vi "draw3.vi"(0 "new position":cluster{"x":i16, "y":i16}, 1 "L 1":dbl(slide)=80.0 scale=0.0..200.0, 2 "L 2":dbl(slide)=80.0 scale=0.0..200.0, 3 "Angle1":dbl(knob)=-45.83837436417874 scale=-90.0..90.0, 4 "Angle 2":dbl(knob)=-72.06882847083946 scale=-90.0..90.0, 5 "input pic in loop":picture, 7 "bias":dbl) -> (14 "end effector":cluster{dbl, dbl}={159.01647214211073, 1.9100783062530127} {"?" format="%.1f"; "?" format="%#.1f"}, 15 "mag":dbl, 16 "angle":dbl, 17 "2D Picture":picture, 18 "shift pic":picture)   [LabVIEW 2024]
panel:
  out "angle3":dbl
  in  "bias 2":dbl
  in  "L 3":dbl(slide)=80.0 scale=0.0..200.0
  # "A 2"
  # "L1"
  # "L2"
  # "A 1"
  # "mm"
  # "mm"
  # "mm"
  # "mm"
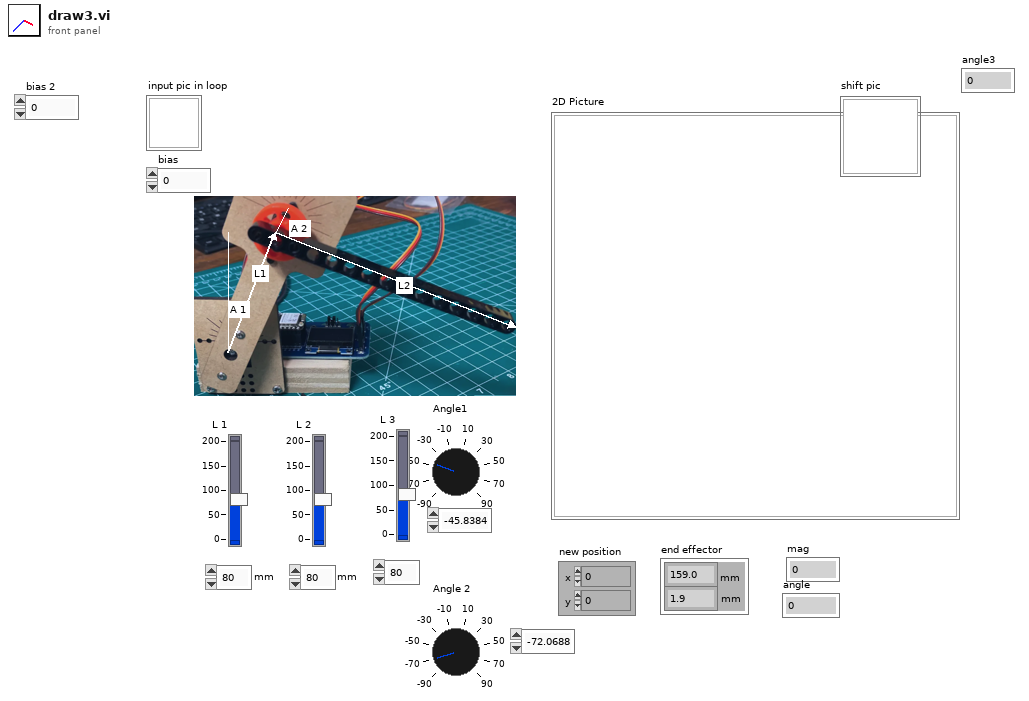
[diagram p1: front panel]
types:
  T1 = cluster{"Width":u16, "Style":enum32{"Solid", "Dash", "Dot", "DashDot", "DashDotDot"}}
  T2 = typedef "imagedata.ctl" = cluster{"image type":i32, "image depth":i32, "image":u8[], "mask":u8[], "colors":u32[], "Rectangle":cluster{"left":i16, "top":i16, "right":i16, "bottom":i16}}
  T3 = cluster{"left":i16, "top":i16, "right":i16, "bottom":i16}
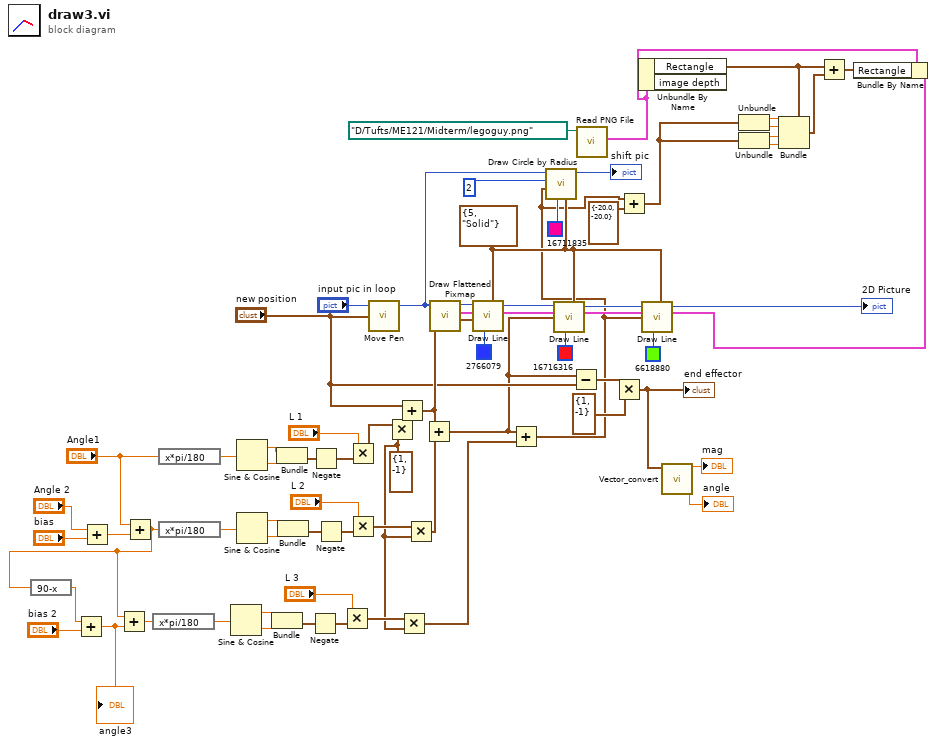
[diagram p0: block diagram]
diagram:
  w25 = cluster{"x":i16, "y":i16} {"x"=1, "y"=-1} ("new position")
  w21 = T1 {"Width"=5, "Style"=enum."Solid"} ("pen")
  n1 = Add(x="Angle 2", y="bias") -> (x+y=w27:dbl)
  n2 = Add(x="Angle1", y=w27) -> (x+y=w18:dbl)
  n3 = expression code="90-x"(w18) -> (w20:dbl)
  n4 = Add(x=w20, y="bias 2") -> (x+y=w29:dbl)
  "angle3" <- w29
  n5 = Add(x=w18, y=w29) -> (x+y=w34:dbl)
  n6 = expression code="x*pi/180"(w34) -> (w35:dbl)
  n7 = expression code="x*pi/180"("Angle1") -> (w68:dbl)
  n8 = expression code="x*pi/180"(w18) -> (w65:dbl)
  n9 = Sine & Cosine(0:w35) -> (1:w32:dbl, 2:w31:dbl)
  n10 = Sine & Cosine(0:w68) -> (1:w55:dbl, 2:w54:dbl)
  n11 = Sine & Cosine(0:w65) -> (1:w52:dbl, 2:w51:dbl)
  n12 = Bundle(w32, w31) -> (w36:cluster{dbl, dbl})  [unwired: 1 in]
  n13 = Bundle(w55, w54) -> (w67:cluster{dbl, dbl})  [unwired: 1 in]
  n14 = Bundle(w52, w51) -> (w66:cluster{dbl, dbl})  [unwired: 1 in]
  n15 = Negate(x=w36) -> (-x=w30:cluster{dbl, dbl})
  n16 = Negate(x=w67) -> (-x=w53:cluster{dbl, dbl})
  n17 = Negate(x=w66) -> (-x=w50:cluster{dbl, dbl})
  n18 = Multiply(x="L 3", y=w30) -> (x*y=w26:cluster{dbl, dbl})
  n19 = Multiply(x="L 1", y=w53) -> (x*y=w40:cluster{dbl, dbl})
  n20 = Multiply(x="L 2", y=w50) -> (x*y=w37:cluster{dbl, dbl})
  n21 = call <vilib>:"Move Pen.vi"("new position"="new position", "picture"="input pic in loop") -> ("new picture"=w5:picture)  [unwired: 3 in]
  n22 = Multiply(x=w40, y=w25) -> (x*y=w39:cluster{dbl, dbl})
  n23 = Add(x="new position", y=w39) -> (x+y=w63:cluster{dbl, dbl})
  n24 = Multiply(x=w26, y=w25) -> (x*y=w24:cluster{dbl, dbl})
  n25 = Multiply(x=w37, y=w25) -> (x*y=w38:cluster{dbl, dbl})
  n26 = Add(x=w38, y=w63) -> (x+y=w19:cluster{dbl, dbl})
  n27 = Add(x=w19, y=w24) -> (x+y=w3:cluster{dbl, dbl})
  n28 = call <vilib>:"Draw Circle by Radius.vi"("pen"=w21, "color(black)"=u32 16711835, "pixel center"=w3, "radius"=u16 2 ("Width"), "picture"=w5) -> ("new picture"=→"shift pic":picture)  [unwired: 6 in]
  n29 = Subtract(x=w19, y="new position") -> (x-y=w58:cluster{dbl, dbl})
  n30 = call <vilib>:"Read PNG File.vi"("path to PNG file"=path "D:/Tufts/ME121/Midterm/legoguy.png") -> ("image data"=w10:T2)  [unwired: 8 in, 2 out]
  n31 = Multiply(x=w58, y=cluster{"x":i16, "y":i16} {"x"=1, "y"=-1} ("new position")) -> (x*y=w49:cluster{dbl, dbl})
  "end effector" <- w49
  n32 = Add(x=w3, y=cluster{dbl, dbl} {-20.0, -20.0} ("x+y")) -> (x+y=w1:cluster{dbl, dbl})
  n33 = Unbundle By Name(w10) -> ("Rectangle"=w7:T3)  [unwired: 1 out]
  n34 = call "Vector_convert.vi"("x,y"=w49) -> ("angle"=→"angle":dbl, "mag"=→"mag":dbl)  [unwired: 9 in]
  n35 = Unbundle(w1) -> (w16:dbl, w15:dbl)
  n36 = Unbundle(w1) -> (w14:dbl, w13:dbl)
  n37 = Bundle(cluster=w7, "left"=w16, "top"=w15, "right"=w14, "bottom"=w13) -> (w8:T3)
  n38 = Add(x=w7, y=w8) -> (x+y=w9:T3)
  n39 = Bundle By Name(cluster=w10, "Rectangle"=w9) -> (w12:T2)
  n40 = call "Draw Flattened Pixmap.vi"("image data"=w12, "picture"=w5) -> ("new picture"=w4:picture)  [unwired: 7 in]
  n41 = call <vilib>:"Draw Line.vi"("picture"=w4, "end point"=w63, "color(black)"=u32 2766079, "pen"=w21) -> ("new picture"=w64:picture)  [unwired: 5 in]
  n42 = call <vilib>:"Draw Line.vi"("picture"=w64, "end point"=w19, "color(black)"=u32 16716316, "pen"=w21) -> ("new picture"=w23:picture)  [unwired: 5 in]
  n43 = call <vilib>:"Draw Line.vi"("picture"=w23, "end point"=w3, "color(black)"=u32 6618880, "pen"=w21) -> ("new picture"=→"2D Picture":picture)  [unwired: 5 in]
